vi "PH_ImageOperator.Position Analysis.vi"(0 "i ref in":refnum<vi>, 5 "error in (no error)":errorcluster) -> (14 "i ref out":refnum<vi>, 19 "error out":errorcluster)   [LabVIEW 2014, in "PH_ImageOperator.lvlib"]
uses:
  PH_ImageOperator.lvlib
  PH_Basics/PH_StatusHandler/PH_StatusHandler.Status.ctl
  PH_Basics/PH_Common/PH_Common.lvlib
  PH_Basics/PH_StatusHandler/PH_StatusHandler.lvlib
panel:
  in  "Case Constant\n(See Context Help)":bool
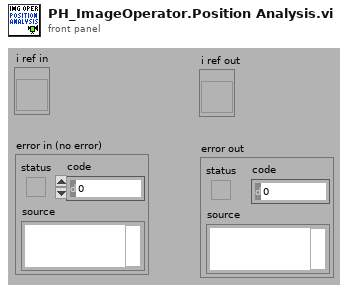
[diagram p1: front panel]
types:
  T1 = typedef "PH_StatusHandler.lvlib/PH_StatusHandler.Status.ctl" = i16
  T2 = typedef "PH_ImageOperator.lvlib/PH_ImageOperator.i attribute.ctl" = cluster{"GUI Refs":cluster{"Delete":refnum<vi>, "Calibration status":refnum<vi>, "BI subtracted":refnum<vi>, "calc Energy":refnum<vi>, "Energy: expected value":refnum<vi>, "Energy: Tolerance":refnum<vi>, "Energy calculated":refnum<vi>, "Energy":refnum<vi>, "calc Beam Anal":refnum<vi>, "Maj Diam 1/esquare":refnum<vi>, "Min Diam 1/esquare":refnum<vi>, "Azi Angle":refnum<vi>, "Min/Maj Diam esquare":refnum<vi>, "Beam analysed":refnum<vi>, "CoG - x":refnum<vi>, "CoG - y":refnum<vi>, "BA: Method":refnum<vi>, "BA: Steps":refnum<vi>, "BA: Factor":refnum<vi>, "calc Traces":refnum<vi>, "Traces: Fit Gauss":refnum<vi>, "Traces calculated":refnum<vi>, "Maj FWHM":refnum<vi>, "Min FWHM":refnum<vi>, "Major Trace":refnum<vi>, "Minor Trace":refnum<vi>, "Maj Fit Order":refnum<vi>, "Min Fit Order":refnum<vi>, "Position calculated":refnum<vi>, "Position":refnum<vi>, "Type":refnum<vi>, "Center":refnum<vi>, "exp - X":refnum<vi>, "exp - Y":refnum<vi>, "Tolerance":refnum<vi>, "f":refnum<vi>, "M":refnum<vi>, "D":refnum<vi>, "q":refnum<vi>, "Dummy Method":refnum<vi>, "Dummy Type":refnum<vi>, "Global On":refnum<vi>, "Traces: No offset":refnum<vi>, "Maj 99%":refnum<vi>, "Min 99%":refnum<vi>, "GUI FF Image":refnum<vi>, "calc Fill Factor":refnum<vi>, "FF calculated":refnum<vi>, "Fill Factor: Filter?":refnum<vi>, "FF: Damage Threshold":refnum<vi>, "FF: Threshold":refnum<vi>, "FF: max allow. Energy":refnum<vi>, "FF: Fillfactor":refnum<vi>, "Calibration data":refnum<vi>}, "List of GUIs":string[], "Calibration":cluster{"Status":T1, "Calibration data":T3, "Calibration Data File":path}, "Final Image":cluster{"BI Subtraction Failure":bool}, "Energy":cluster{"on":bool, "expected value [mJ]":dbl, "Tolerance [%]":dbl, "State":T1, "Energy [mJ]":dbl, "Unit":string, "calculated @":timestamp}, "Beam Analysis":cluster{"on":bool, "Data":T4, "Method":bool, "Steps":i32, "Factor":i32, "ROI":cluster{"Left":i32, "Top":i32, "Right":i32, "Bottom":i32}, "analysed @":timestamp}, "Trace Analysis":cluster{"on":bool, "Fit on":bool, "Maj FWHM":dbl, "Min FWHM":dbl, "Maj Fit Order":i32, "Min Fit Order":i32, "No Offset":bool, "Maj 99%":dbl, "Min 99%":dbl, "Traces":cluster{"XScaleName":string, "Y Scale Minimum":sgl, "Y Scale Maximum":sgl, "X Scale Minimum":sgl, "X Scale Maximum":sgl, "Traces":cluster{"Index":sgl[], "Trace":dbl[]}[]}[], "analysed @":timestamp}, "Position Analysis":cluster{"on":bool, "exp - X":i32, "exp - Y":i32, "focal length [mm]":dbl, "Magnification":dbl, "Delta":dbl, "Theta":dbl, "Tolerance":dbl, "Type":bool, "analysed @":timestamp}, "Fill Factor":cluster{"on":bool, "Filter on?":bool, "Threshold":dbl, "Damage Threshold [J/cm²]":dbl, "Fillfactor":dbl, "Max. allowed Energy [J]":dbl, "calculated @":timestamp}, "Statistician Service ID":i32, "Images":cluster{"Background":T5, "OP":T5, "GUI":T5, "BA: ROI":T5, "Trace: Turn":T5, "FF: Main":T5, "FF: Help":T5, "PSDB: BG":T5, "PSDB: OP":T5, "PSDB: FF":T5}}
  T3 = typedef "PH_ImageCalibrator.lvlib/PH_ImageCalibrator.Calibration Data.ctl" = cluster{"Date":string, "Time":string, "Cam Settings":cluster{"Cam ID":string, "Gain":dbl, "Brightness":dbl, "Shutter":dbl, "Cam Error":bool, "Mode":i32}, "Background Image":cluster{"Image":dbl[][], "Image Error":bool}, "Linear Calibration":cluster{"Calibration Factor":dbl, "not mm or mrad":bool}, "Energy Calibration":cluster{"Calibration Factor":dbl, "no mJ":bool}}
  T4 = typedef "PH_ImageOperator.lvlib/PH_ImageOperator.Beam Analysis Data.ctl" = cluster{"CoG-x":sgl, "CoG-y":sgl, "Maj Dim":dbl, "Min Dim":dbl, "Ellipticity":dbl, "Azimuth Angle [rad]":dbl, "Azi Angle rel to Maj?":bool}
  T5 = typedef "IMAQ Image.ctl" = refnum<image>
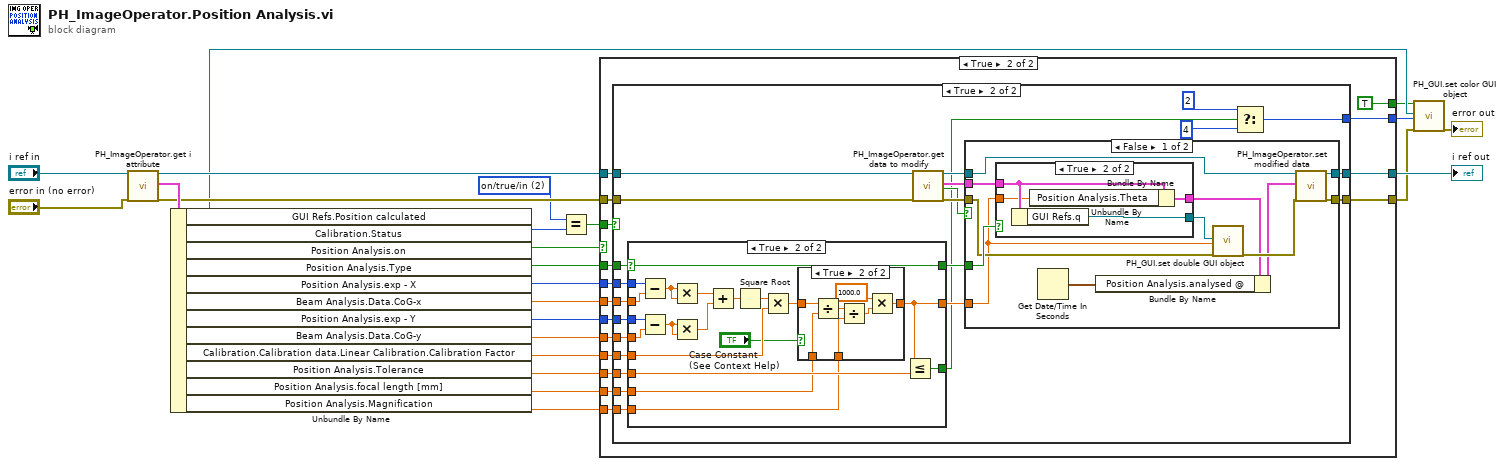
[diagram p0: block diagram]
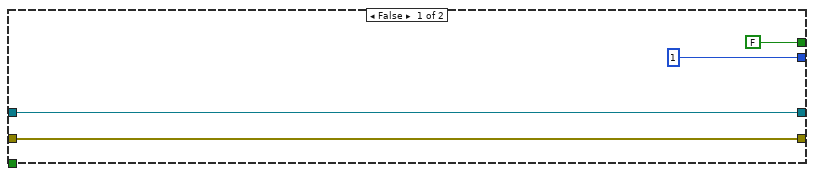
[diagram p2: hidden frame]
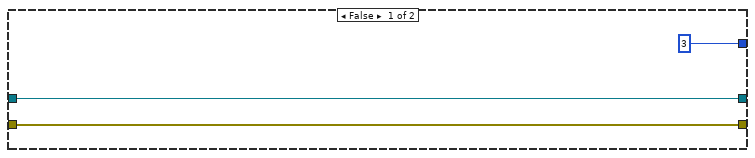
[diagram p3: hidden frame]
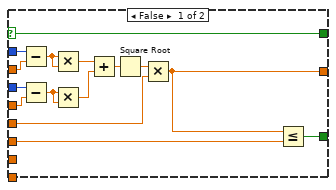
[diagram p4: hidden frame]
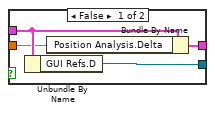
[diagram p6: hidden frame]
diagram:
  w11 = T1 2 items=["no info", "off/false/out", "on/true/in", "Failure", "Alarm", "Status 1", "Status 2", "Status 3"] ("Calibration.Status")
  n1 = call "PH_ImageOperator.get i attribute.vi"("i ref in"="i ref in", "error in (no error)"="error in (no error)") -> ("i ref out"=w20:refnum<vi>, "i attribute"=w22:T2, "error out"=w21:errorcluster)  [unwired: 15 in]
  n2 = Unbundle By Name(w22) -> ("GUI Refs.Position calculated"=w7:refnum<vi>, "Calibration.Status"=w12:T1, "Position Analysis.on"=w18:bool, "Position Analysis.Type"=w17:bool, "Position Analysis.exp - X"=w15:i32, "Beam Analysis.Data.CoG-x"=w16:sgl, "Position Analysis.exp - Y"=w14:i32, "Beam Analysis.Data.CoG-y"=w13:sgl, "Calibration.Calibration data.Linear Calibration.Calibration Factor"=w5:dbl, "Position Analysis.Tolerance"=w4:dbl, "Position Analysis.focal length [mm]"=w3:dbl, "Position Analysis.Magnification"=w2:dbl)
  n3 = Equal?(x=w11, y=w12) -> (x = y?=w10:bool)
  n4 = case shown="True" w18 {
    tunnel: w21 -> [w27 w44]
    tunnel: [w27 w43] -> w8
    tunnel: w20 -> [w28 w42]
    tunnel: [w28 w41] -> w19
    tunnel: w17 -> [_ w40]
    tunnel: w16 -> [_ w39]
    tunnel: w15 -> [_ w38]
    tunnel: w14 -> [_ w37]
    tunnel: w13 -> [_ w36]
    tunnel: w10 -> [_ w35]
    tunnel: [1 w34] -> w6
    tunnel: w5 -> [_ w33]
    tunnel: w4 -> [_ w32]
    tunnel: w3 -> [_ w31]
    tunnel: w2 -> [_ w30]
    tunnel: [FALSE TRUE] -> w1
    frame False {
    }
    frame True {
      n5 = case shown="True" w35 {
        tunnel: w44 -> [w46 w68]
        tunnel: [w46 w67] -> w43
        tunnel: w42 -> [w45 w66]
        tunnel: [w45 w65] -> w41
        tunnel: w40 -> [_ w62]
        tunnel: w39 -> [_ w60]
        tunnel: w38 -> [_ w59]
        tunnel: w37 -> [_ w58]
        tunnel: w36 -> [_ w57]
        tunnel: [3 w51] -> w34
        tunnel: w33 -> [_ w56]
        tunnel: w32 -> [_ w54]
        tunnel: w31 -> [_ w49]
        tunnel: w30 -> [_ w48]
        frame False {
        }
        frame True {
          n6 = case shown="True" w62 {
            selector: w62 -> [w85 w104]
            tunnel: [w85 w104] -> w61
            tunnel: w60 -> [w83 w102]
            tunnel: w59 -> [w84 w103]
            tunnel: w58 -> [w82 w101]
            tunnel: w57 -> [w81 w100]
            tunnel: w56 -> [w74 w93]
            tunnel: [w73 w87] -> w55
            tunnel: w54 -> [w72 w92]
            tunnel: [w71 w91] -> w50
            tunnel: w49 -> [_ w90]
            tunnel: w48 -> [_ w89]
            frame False {
              n7 = Subtract(x=w84, y=w83) -> (x-y=w80:sgl)
              n8 = Subtract(x=w82, y=w81) -> (x-y=w79:sgl)
              n9 = Multiply(x=w80, y=w80) -> (x*y=w78:sgl)
              n10 = Multiply(x=w79, y=w79) -> (x*y=w77:sgl)
              n11 = Add(x=w78, y=w77) -> (x+y=w76:sgl)
              n12 = Square Root(x=w76) -> (sqrt(x)=w75:sgl)
              n13 = Multiply(x=w75, y=w74) -> (x*y=w73:dbl)
              n14 = Less Or Equal?(x=w73, y=w72) -> (x <= y?=w71:bool)
            }
            frame True {
              n15 = Subtract(x=w103, y=w102) -> (x-y=w99:sgl)
              n16 = Subtract(x=w101, y=w100) -> (x-y=w98:sgl)
              n17 = Multiply(x=w99, y=w99) -> (x*y=w97:sgl)
              n18 = Multiply(x=w98, y=w98) -> (x*y=w96:sgl)
              n19 = Add(x=w97, y=w96) -> (x+y=w95:sgl)
              n20 = Square Root(x=w95) -> (sqrt(x)=w94:sgl)
              n21 = Multiply(x=w94, y=w93) -> (x*y=w88:dbl)
              n22 = case shown="True" "Case Constant\n(See Context Help)" {
                tunnel: w90 -> [_ w112]
                tunnel: w89 -> [_ w110]
                tunnel: w88 -> [w105 w109]
                tunnel: [w105 w106] -> w87
                frame False {
                }
                frame True {
                  n23 = Divide(x=w109, y=w112) -> (x/y=w111:dbl)
                  n24 = Divide(x=w111, y=w110) -> (x/y=w107:dbl)
                  n25 = Multiply(x=1000.0, y=w107) -> (x*y=w106:dbl)
                }
              }
              n26 = Less Or Equal?(x=w87, y=w92) -> (x <= y?=w91:bool)
            }
          }
          n27 = call "PH_ImageOperator.get data to modify.vi"("i ref in"=w66, "error in (no error)"=w68) -> ("i ref out"=w69:refnum<vi>, "i attribute"=w63:T2, "timed out"=w64:bool, "error out"=w70:errorcluster)  [unwired: 14 in]
          n28 = case shown="False" w64 {
            tunnel: w70 -> [w117 w133]
            tunnel: w69 -> [w118 w134]
            tunnel: [w124 w133] -> w67
            tunnel: [w123 w134] -> w65
            tunnel: w63 -> [w122 _]
            tunnel: w55 -> [w116 _]
            tunnel: w61 -> [w121 _]
            frame False {
              n29 = case shown="True" w121 {
                tunnel: [w128 w132] -> w114
                tunnel: w122 -> [w127 w131]
                tunnel: [w126 w130] -> w120
                tunnel: w116 -> [w125 w129]
                frame False {
                  n30 = Unbundle By Name(w127) -> ("GUI Refs.D"=w126:refnum<vi>)
                  n31 = Bundle By Name(cluster=w127, "Position Analysis.Delta"=w125) -> (w128:T2)
                }
                frame True {
                  n32 = Unbundle By Name(w131) -> ("GUI Refs.q"=w130:refnum<vi>)
                  n33 = Bundle By Name(cluster=w131, "Position Analysis.Theta"=w129) -> (w132:T2)
                }
              }
              n34 = Get Date/Time In Seconds() -> (seconds since 1Jan1904=w113:timestamp)
              n35 = Bundle By Name(cluster=w114, "Position Analysis.analysed @"=w113) -> (w115:T2)
              n36 = call "PH_GUI.set double GUI object.vi"("GUI object Ref"=w120, "value"=w116, "error in (no error)"=w117) -> ("error out"=w119:errorcluster)  [unwired: 16 in]
              n37 = call "PH_ImageOperator.set modified data.vi"("i ref in"=w118, "i attribute"=w115, "error in (no error)"=w119) -> ("i ref out"=w123:refnum<vi>, "error out"=w124:errorcluster)  [unwired: 15 in]
            }
            frame True {
            }
          }
          n38 = Select(t=2, s=w50, f=4) -> (s? t:f=w51:i32)
        }
      }
    }
  }
  "i ref out" <- w19
  n39 = call "PH_GUI.set color GUI object.vi"("Visible? (true)"=w1, "GUI object Ref"=w7, "State"=w6, "error in (no error)"=w8) -> ("error out"=→"error out":errorcluster)  [unwired: 15 in]
